vi "Collect Data2D.vi"(8 "error in (no error)":errorcluster, 10 "Data2D in":refnum<class "Data2D.lvclass">, 11 "AverageCollector2D in":refnum<class "AverageCollector2D.lvclass">) -> (0 "error out":errorcluster, 2 "finished?":bool=TRUE, 3 "AverageCollector2D out":refnum<class "AverageCollector2D.lvclass">)   [LabVIEW 2014, in "AverageCollector2D.lvclass"]
uses:
  AverageCollector2D.lvclass
  Framework/Model/Data/Data2D/Data2D.lvclass
  Framework/Collector/AbstractCollector/AbstractCollector.lvclass/AbstractCollector.ctl
  Framework/Collector/AbstractCollector/AbstractCollector.lvclass
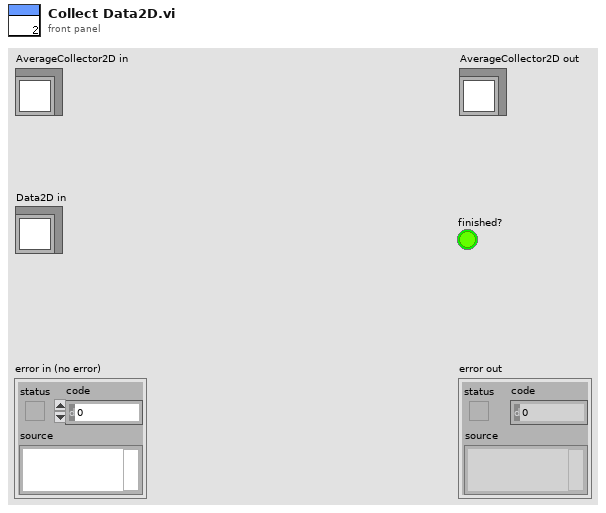
[diagram p1: front panel]
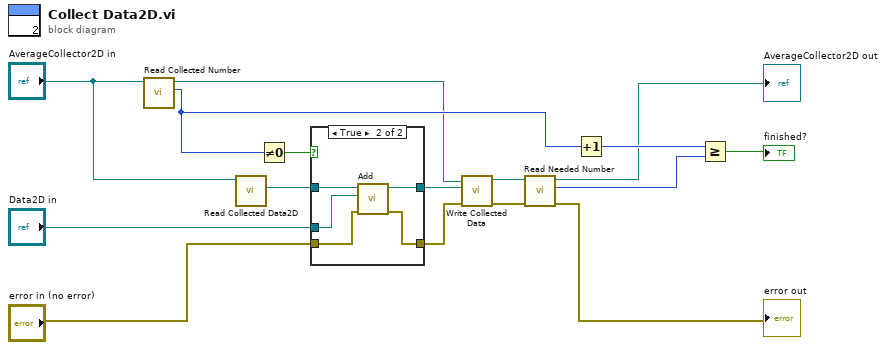
[diagram p0: block diagram]
diagram:
  n1 = call "Read Collected Number.vi"("AbstractCollector in"="AverageCollector2D in") -> ("collected"=w15:u32, "AbstractCollector out"=w8:refnum<class "AverageCollector2D.lvclass">)  [unwired: 8 in, 1 out]
  n2 = call-dynamic "Read Collected Data2D.vi"("AbstractCollector2D in"="AverageCollector2D in") -> ("Collected Data"=w1:refnum<class "Data2D.lvclass">)  [unwired: 8 in, 2 out]
  n3 = Not Equal To 0?(x=w15) -> (x != 0?=w14:bool)
  n4 = case shown="True" w14 {
    tunnel: [w17 w23] -> w13
    tunnel: [w18 w20] -> w12
    tunnel: "error in (no error)" -> [w18 w21]
    tunnel: w1 -> [_ w19]
    tunnel: "Data2D in" -> [w17 w22]
    frame False {
    }
    frame True {
      n5 = call-dynamic "Add.vi"("error in (no error)"=w21, "Data2D 2"=w22, "Data2D in"=w19) -> ("error out"=w20:errorcluster, "Data2D out"=w23:refnum<class "Data2D.lvclass">)  [unwired: 7 in]
    }
  }
  n6 = call-dynamic "Write Collected Data.vi"("error in (no error)"=w12, "Collected Data"=w13, "AbstractCollector in"=w8) -> ("error out"=w9:errorcluster, "AbstractCollector out"=w11:refnum<class "AverageCollector2D.lvclass">)  [unwired: 7 in]
  n7 = call-dynamic "Read Needed Number.vi"("error in (no error)"=w9, "AbstractCollector in"=w11) -> ("error out"=→"error out":errorcluster, "Needed Number"=w10:u32, "AbstractCollector out"=→"AverageCollector2D out":refnum<class "AverageCollector2D.lvclass">)  [unwired: 7 in]
  n8 = Increment(x=w15) -> (x+1=w16:u32)
  n9 = Greater Or Equal?(x=w16, y=w10) -> (x >= y?=→"finished?":bool)
